vi "Add Local.vi"(6 "Parent":string[](array[string]), 7 "Type":T1, 8 "error in (no error)":errorcluster, 9 "Value":string, 10 "Name":string, 11 "TemplateLocals in":refnum<class "Value Tree.lvclass">) -> (0 "error out":errorcluster, 3 "TemplateLocals out":refnum<class "Value Tree.lvclass">, 4 "Hierarchy":string[](array[string]))   [LabVIEW 2020, in "HTTP Server.lvlib" / "Value Tree.lvclass"]
uses:
  Value Tree.lvclass
  Local Type.ctl
  Value Tree.lvclass/Value Tree.ctl
  Local Info.ctl
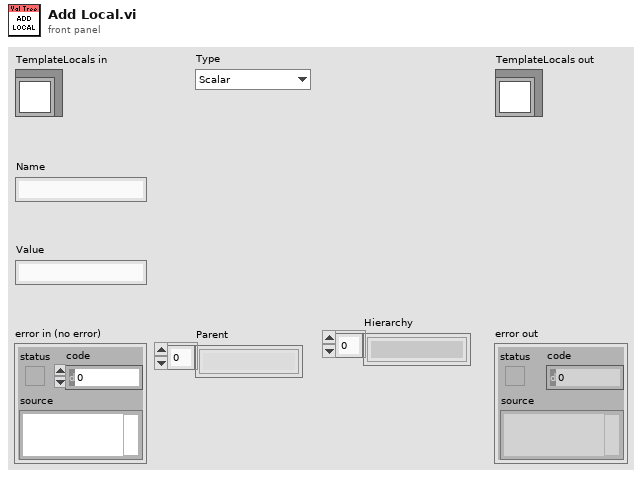
[diagram p1: front panel]
types:
  T1 = typedef "HTTP Server.lvlib/Value Tree.lvclass/Local Type.ctl" = enum16{"Scalar", "Object", "Array"}
  T2 = typedef "HTTP Server.lvlib/Value Tree.lvclass/Local Info.ctl" = cluster{"Type":T1, "Value":string, "Children":string[], "Size":i32}
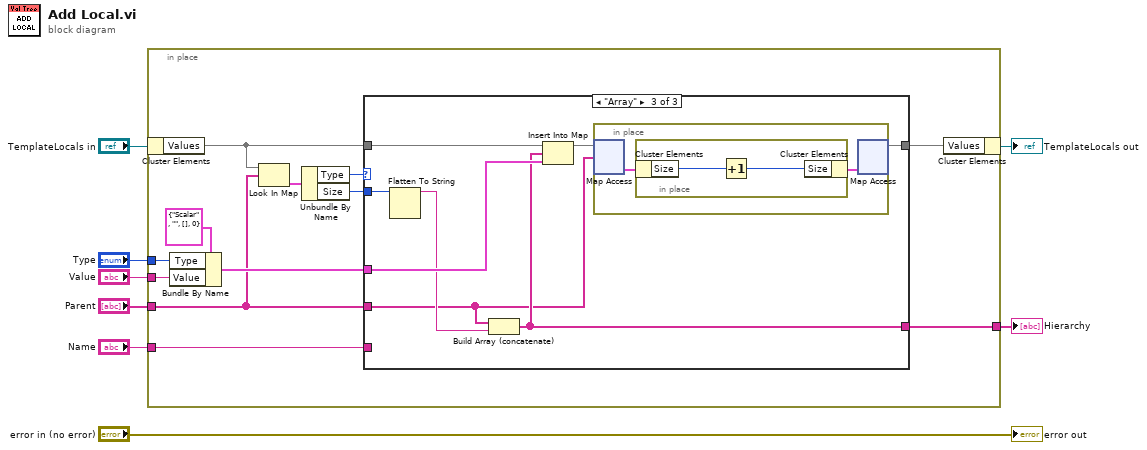
[diagram p0: block diagram]
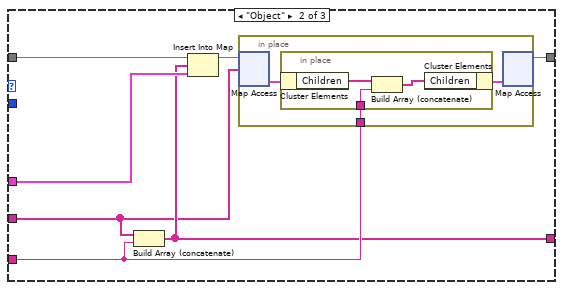
[diagram p3: hidden frame]
diagram:
  n1 = in-place {
    in-place-border: "Value" -> [w16]
    in-place-border: "Type" -> [w17]
    in-place-border: "Parent" -> [w14]
    in-place-border: "Name" -> [w13]
    in-place-border: [w12] -> w1
    n2 = in-place-cluster #1("TemplateLocals in") -> ("Values"=w19:map{string[], T2})
    n3 = Bundle By Name(cluster=T2 {"Type"=enum."Scalar", "Value"="", "Children"=[], "Size"=0} ("Local Info"), "Type"=w17, "Value"=w16) -> (w15:T2)
    n4 = Look In Map(map=w19, key=w14) -> (value=w11:T2)  [unwired: 1 in, 1 out]
    n5 = Unbundle By Name(w11) -> ("Type"=w10:T1, "Size"=w9:i32)
    n6 = case shown="\"Array\"" w10 {
      tunnel: [w21 w28 w42] -> w20
      tunnel: w19 -> [w21 w26 w40]
      tunnel: w15 -> [_ w25 w39]
      tunnel: w14 -> [_ w22 w35]
      tunnel: w13 -> [_ w24 _]
      tunnel: w9 -> [_ _ w37]
      tunnel: [_ w23 w38] -> w12
      frame "Scalar" {
      }
      frame "Object" {
        n7 = Build Array (concatenate)(w22, w24) -> (w23:string[])
        n8 = Insert Into Map(map in=w26, key=w23, value=w25) -> (map out=w27:map{string[], T2})  [unwired: 2 out]
        n9 = in-place {
          in-place-border: w24 -> [w29]
          n10 = in-place-map #2(w27, w22) -> (w31:T2)  [unwired: 1 in, 1 out]
          n11 = in-place {
            in-place-border: w29 -> [w33]
            n12 = in-place-cluster #3(w31) -> ("Children"=w34:string[])
            n13 = Build Array (concatenate)(w34, w33) -> (w32:string[])
            n14 = in-place-cluster #3("Children"=w32) -> (w30:T2)
          }
          n15 = in-place-map #2(w30) -> (w28:map{string[], T2})  [unwired: 1 in, 2 out]
        }
      }
      frame "Array" {
        n16 = Flatten To String(anything=w37) -> (data string=w36:string)  [unwired: 3 in, 2 out]
        n17 = Build Array (concatenate)(w35, w36) -> (w38:string[])
        n18 = Insert Into Map(map in=w40, key=w38, value=w39) -> (map out=w41:map{string[], T2})  [unwired: 2 out]
        n19 = in-place {
          n20 = in-place-map #4(w41, w35) -> (w44:T2)  [unwired: 1 in, 1 out]
          n21 = in-place {
            n22 = in-place-cluster #5(w44) -> ("Size"=w46:i32)
            n23 = Increment(x=w46) -> (x+1=w45:i32)
            n24 = in-place-cluster #5("Size"=w45) -> (w43:T2)
          }
          n25 = in-place-map #4(w43) -> (w42:map{string[], T2})  [unwired: 1 in, 2 out]
        }
      }
    }
    n26 = in-place-cluster #1("Values"=w20) -> (→"TemplateLocals out":refnum<class "Value Tree.lvclass">)
  }
  "Hierarchy" <- w1
  "error out" <- "error in (no error)"
